vi "Kei2400 Current.vi"(5 "Exec":bool, 6 "VISA resource name":refnum<visa-resource-name>="GPIB0::26::INSTR", 7 "Init":bool, 8 "error in (no error)":errorcluster, 11 "Current mA":dbl=10.0) -> (0 "error out":errorcluster)   [LabVIEW 2024]
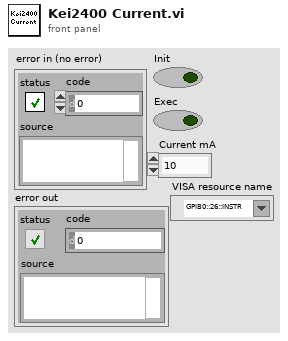
[diagram p1: front panel]
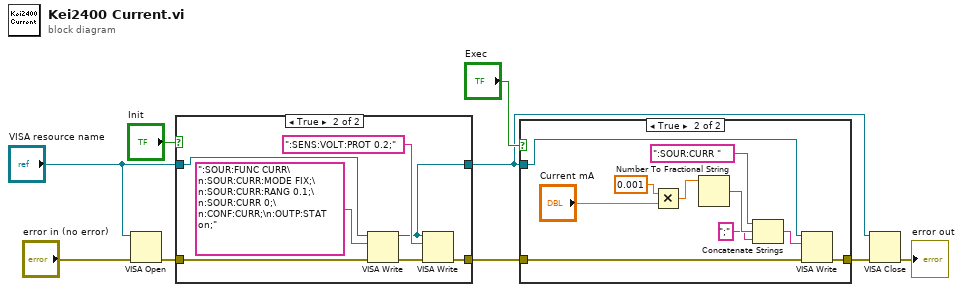
[diagram p0: block diagram]
diagram:
  n1 = VISA Open(error in (no error)="error in (no error)", VISA resource name="VISA resource name") -> (error out=w4:errorcluster)  [unwired: 3 in, 1 out]
  n2 = case shown="True" "Init" {
    tunnel: w4 -> [w11 w18]
    tunnel: "VISA resource name" -> [w10 w17]
    tunnel: [w11 w15] -> w7
    tunnel: [w10 w13] -> w1
    frame False {
    }
    frame True {
      n3 = VISA Write(VISA resource name=w17, write buffer=":SOUR:FUNC CURR\n:SOUR:CURR:MODE FIX;\n:SOUR:CURR:RANG 0.1;\n:SOUR:CURR 0;\n:CONF:CURR;\n:OUTP:STAT on;", error in (no error)=w18) -> (VISA resource name out=w13:refnum<visa-resource-name>, error out=w12:errorcluster)  [unwired: 1 out]
      n4 = VISA Write(VISA resource name=w13, write buffer=":SENS:VOLT:PROT 0.2;", error in (no error)=w12) -> (error out=w15:errorcluster)  [unwired: 2 out]
    }
  }
  n5 = case shown="True" "Exec" {
    tunnel: w7 -> [w19 w27]
    tunnel: w1 -> [_ w25]
    tunnel: [w19 w26] -> w3
    frame False {
    }
    frame True {
      n6 = Multiply(x=0.001, y="Current mA") -> (x*y=w24:dbl)
      n7 = Number To Fractional String(number=w24) -> (F-format string=w22:string)  [unwired: 3 in]
      n8 = Concatenate Strings(":SOUR:CURR " ("string"), w22, ";" ("string")) -> (w20:string)
      n9 = VISA Write(VISA resource name=w25, write buffer=w20, error in (no error)=w27) -> (error out=w26:errorcluster)  [unwired: 2 out]
    }
  }
  n10 = VISA Close(VISA resource name=w1, error in (no error)=w3) -> (error out=→"error out":errorcluster)
